vi "Set Chassis Timing Source.vi"(8 "error in (no error)":errorcluster, 10 "Timing Source":enum16{"Automatic", "Custom Device"}(ring), 11 "Item Ref in":T1 format="%.0x") -> (0 "error out":errorcluster, 3 "Item Ref out":T1 format="%.0x")   [LabVIEW 2010, in "PXIe-433x Custom Device.lvlib"]
uses:
  PXIe-433x Custom Device.lvlib
  <vilib>/NI Veristand/Custom Device API/Custom Device Item Ref.ctl
  NationalInstruments.VeriStand.SystemStorage
  <vilib>/NI Veristand/Custom Device API/Custom Device API.lvlib
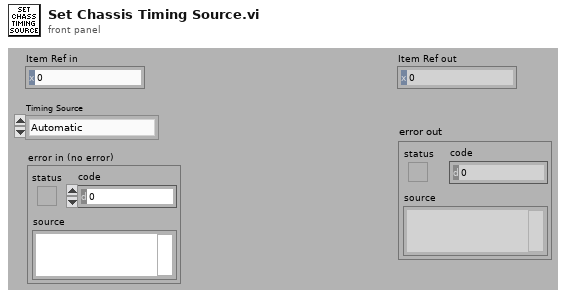
[diagram p1: front panel]
types:
  T1 = typedef "Custom Device API.lvlib/Custom Device Item Ref.ctl" = u64
  T2 = typedef "Custom Device API.lvlib/Custom Device Pointer.ctl" = refnum<k24>
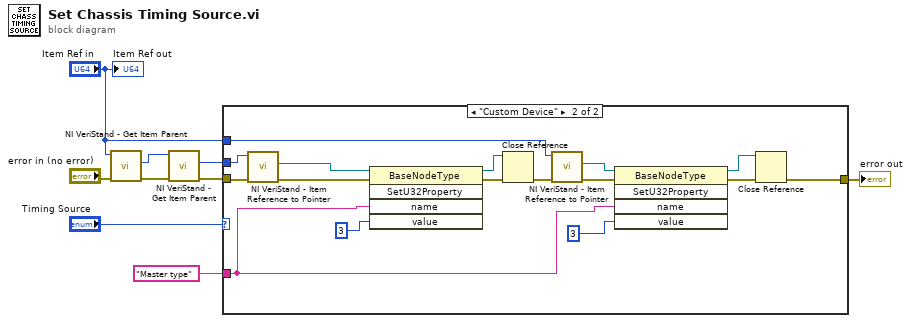
[diagram p0: block diagram]
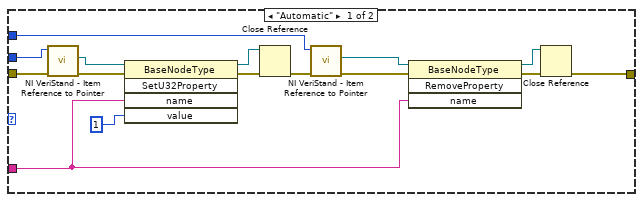
[diagram p2: hidden frame]
diagram:
  n1 = call <vilib>:"NI VeriStand - Get Item Parent.vi"("error in (no error)"="error in (no error)", "Item Ref in"="Item Ref in") -> ("error out"=w5:errorcluster, "Parent Ref"=w6:T1)  [unwired: 6 in, 2 out]
  n2 = call <vilib>:"NI VeriStand - Get Item Parent.vi"("error in (no error)"=w5, "Item Ref in"=w6) -> ("error out"=w4:errorcluster, "Parent Ref"=w3:T1)  [unwired: 6 in, 2 out]
  n3 = case shown="\"Custom Device\"" "Timing Source" {
    tunnel: [w10 w26] -> w9
    tunnel: w4 -> [w19 w37]
    tunnel: w3 -> [w18 w36]
    tunnel: "Item Ref in" -> [w14 w32]
    tunnel: "Master type" ("name") -> [w11 w25]
    frame "Automatic" {
      n4 = call <vilib>:"NI VeriStand - Item Reference to Pointer.vi"("error in (no error)"=w19, "Item Ref in"=w18) -> ("error out"=w24:errorcluster, "Node Pointer"=w23:T2)  [unwired: 6 in, 2 out]
      n5 = invoke class="BaseNodeType" method="SetU32Property"(reference=w23, error in=w24, "name"=w11, "value"=u32 1) -> (reference out=w16:T2, error out=w17:errorcluster)  [unwired: 1 in, 3 out]
      n6 = Close Reference(reference=w16, error in (no error)=w17) -> (error out=w15:errorcluster)
      n7 = call <vilib>:"NI VeriStand - Item Reference to Pointer.vi"("error in (no error)"=w15, "Item Ref in"=w14) -> ("error out"=w13:errorcluster, "Node Pointer"=w12:T2)  [unwired: 6 in, 2 out]
      n8 = invoke class="BaseNodeType" method="RemoveProperty"(reference=w12, error in=w13, "name"=w11) -> (reference out=w21:T2, error out=w20:errorcluster)  [unwired: 1 in, 2 out]
      n9 = Close Reference(reference=w21, error in (no error)=w20) -> (error out=w10:errorcluster)
    }
    frame "Custom Device" {
      n10 = call <vilib>:"NI VeriStand - Item Reference to Pointer.vi"("error in (no error)"=w37, "Item Ref in"=w36) -> ("error out"=w38:errorcluster, "Node Pointer"=w40:T2)  [unwired: 6 in, 2 out]
      n11 = invoke class="BaseNodeType" method="SetU32Property"(reference=w40, error in=w38, "name"=w25, "value"=u32 3) -> (reference out=w34:T2, error out=w35:errorcluster)  [unwired: 1 in, 3 out]
      n12 = Close Reference(reference=w34, error in (no error)=w35) -> (error out=w33:errorcluster)
      n13 = call <vilib>:"NI VeriStand - Item Reference to Pointer.vi"("error in (no error)"=w33, "Item Ref in"=w32) -> ("error out"=w31:errorcluster, "Node Pointer"=w30:T2)  [unwired: 6 in, 2 out]
      n14 = invoke class="BaseNodeType" method="SetU32Property"(reference=w30, error in=w31, "name"=w25, "value"=u32 3) -> (reference out=w27:T2, error out=w28:errorcluster)  [unwired: 1 in, 3 out]
      n15 = Close Reference(reference=w27, error in (no error)=w28) -> (error out=w26:errorcluster)
    }
  }
  "error out" <- w9
  "Item Ref out" <- "Item Ref in"
